vi "反馈节点 与 反馈节点子vi.vi"() -> ()   [LabVIEW 2023]
panel:
  out "Array 5":dbl[](array[numeric])
  out "Array 6":dbl[](array[numeric])
  out "Array 4":dbl[](array[numeric])
  out "Array 3":dbl[](array[numeric])
  out "Array 2":dbl[](array[numeric])
  out "Array":dbl[](array[numeric])
  # "反馈节点4"
  # "如果 把反馈 节点 变成 一个 子vi 那么 引用的时候， \n这些 子 vi 共享一个 寄存器。。。WTF！！！！"
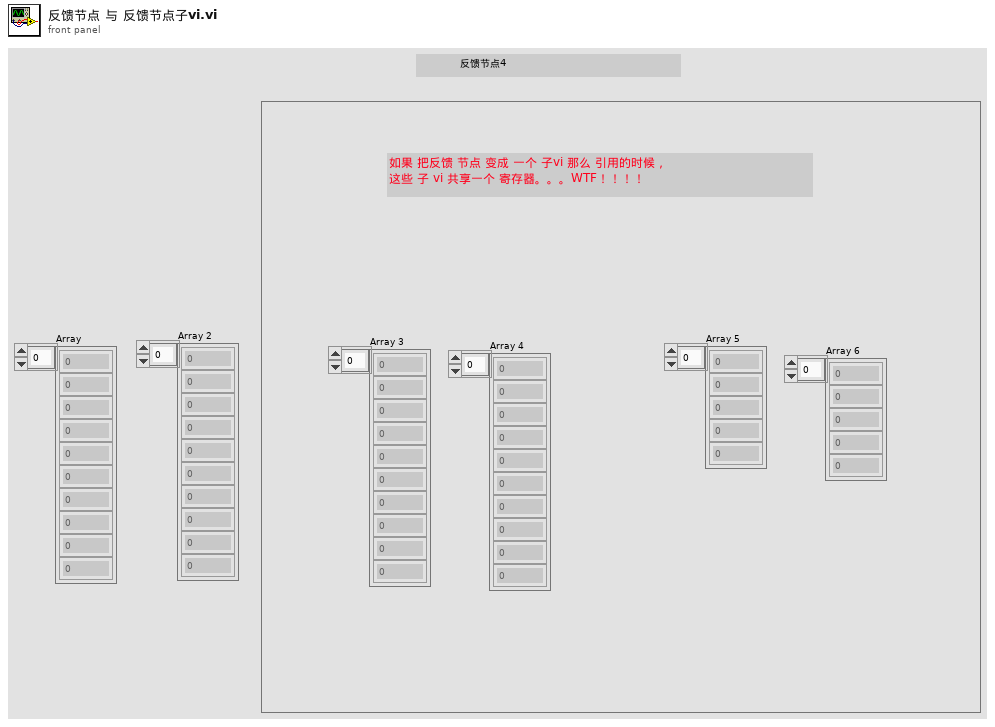
[diagram p1: front panel]
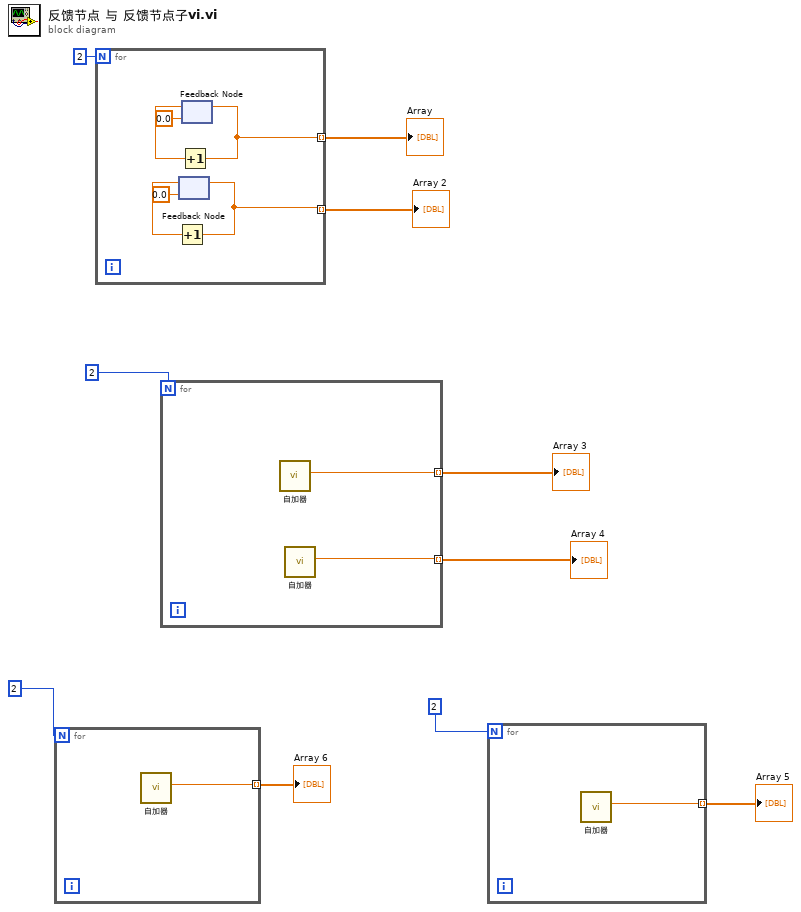
[diagram p0: block diagram]
diagram:
  n1 = for {
    N: 2 -> [_]
    tunnel: [w11] -> w4 mode=indexing
    n2 = call "自加器.vi"() -> ("output"=w11:dbl)  [unwired: 11 in]
  }
  "Array 6" <- w4
  n3 = for {
    N: 2 -> [_]
    tunnel: [w15] -> w10 mode=indexing
    tunnel: [w12] -> w9 mode=indexing
    n4 = feedback #1(0.0) -> (w14:dbl)
    n5 = Increment(x=w14) -> (x+1=w12:dbl)
    n6 = feedback-in #1(w12) -> ()
    n7 = feedback #2(0.0) -> (w17:dbl)
    n8 = Increment(x=w17) -> (x+1=w15:dbl)
    n9 = feedback-in #2(w15) -> ()
  }
  "Array" <- w10
  "Array 2" <- w9
  n10 = for {
    N: 2 -> [_]
    tunnel: [w19] -> w7 mode=indexing
    tunnel: [w18] -> w6 mode=indexing
    n11 = call "自加器.vi"() -> ("output"=w19:dbl)  [unwired: 11 in]
    n12 = call "自加器.vi"() -> ("output"=w18:dbl)  [unwired: 11 in]
  }
  "Array 3" <- w7
  "Array 4" <- w6
  n13 = for {
    N: 2 -> [_]
    tunnel: [w20] -> w2 mode=indexing
    n14 = call "自加器.vi"() -> ("output"=w20:dbl)  [unwired: 11 in]
  }
  "Array 5" <- w2
